vi "ADCP_write_parameter_to_serial_port_emulator_queue.vi"(0 "ADCP In":refnum<class "ADCP.lvclass">, 5 "Parameter Name":string, 7 "Parameter Value":string, 11 "error in (no error)":errorcluster) -> (4 "ADCP out":refnum<class "ADCP.lvclass">, 6 "Queue Out":refnum<queue>, 15 "error out":errorcluster)   [LabVIEW 2017, in "ADCP.lvclass"]
uses:
  ADCP.lvclass
  ADCP.lvclass/ADCP.ctl
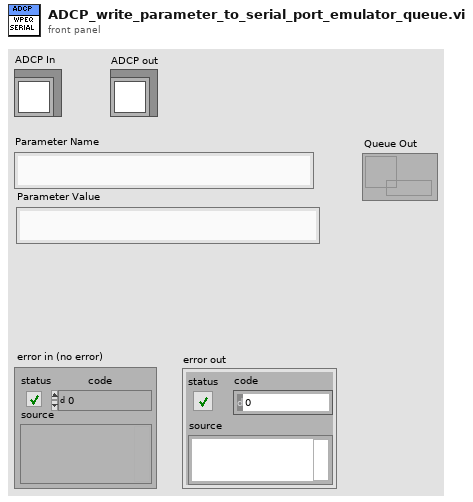
[diagram p1: front panel]
types:
  T1 = typedef "ADCP.lvclass/ADCP_Data_Packet_Transmit_Mode.ctl" = enum16{"Disable", "Single", "Cyclic", "Repeat"}
  T2 = cluster{"Parameters":cluster{"Parameter name":string, "Node name":string, "Node ID":u8, "Frame name":string, "Frame ID":u8, "Start bit":u32, "Bit length":u32, "Factor":dbl, "Offset":dbl, "Minimum":dbl, "Maximum":dbl, "Value":string, "Comments":string, "Data_Type":enum16{"BOOL", "UNSIGNED", "SIGNED", "FLOAT32", "ENUM"}, "Enum List":string[]}[], "Priority":enum16{"LOW", "HIGH"}, "Node name":string, "Node ID":u8, "Frame name":string, "Frame ID":u8, "Data":u32, "Raw bytes":u8[], "Processed bytes":u8[], "Tx count":i32, "Last Tx Time":u32, "Tx interval":u32, "Rx count":i32, "Last Rx Time":u32, "Rx interval":u32, "Tx Enable":bool, "Tx mode":T1, "Repeat/Cyclic Tx interval":u32, "Repeat count":u16}
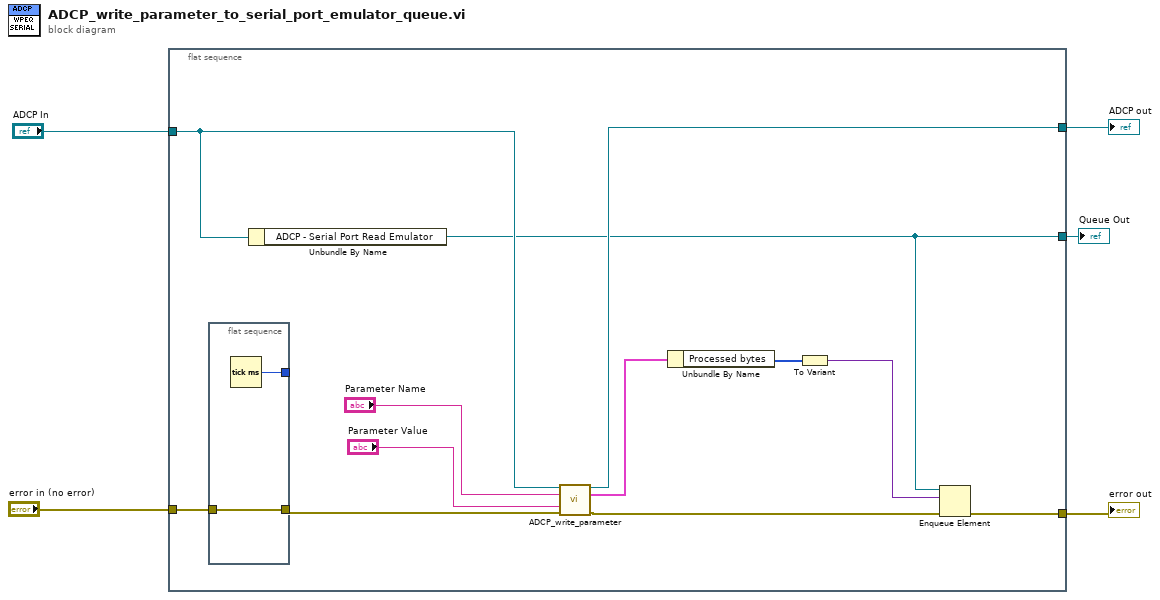
[diagram p0: block diagram]
diagram:
  n1 = flat-sequence {
    tunnel: "ADCP In" -> [w15]
    tunnel: "error in (no error)" -> [w17]
    tunnel: [w8] -> w3
    tunnel: [w7] -> w2
    tunnel: [w6] -> w1
    frame #0 {
      n2 = flat-sequence {
        tunnel: w17 -> [w19]
        tunnel: [w19] -> w16
        tunnel: [w18] -> _
        frame #0 {
          n3 = Tick Count (ms)() -> (millisecond timer value=w18:u32)
        }
      }
      n4 = Unbundle By Name(w15) -> ("ADCP - Serial Port Read Emulator"=w6:refnum<queue>)
      n5 = call "ADCP_write_parameter.vi"("ADCP in"=w15, "Parameter Name"="Parameter Name", "Parameter Value"="Parameter Value", "error in (no error)"=w16) -> ("ADCP out"=w7:refnum<class "ADCP.lvclass">, "Data Packet out"=w12:T2, "error out"=w10:errorcluster)  [unwired: 9 in]
      n6 = Unbundle By Name(w12) -> ("Processed bytes"=w11:u8[])
      n7 = To Variant(anything=w11) -> (Variant=w9:variant)
      n8 = Enqueue Element(queue=w6, element=w9, error in (no error)=w10) -> (error out=w8:errorcluster)  [unwired: 1 in, 2 out]
    }
  }
  "error out" <- w3
  "ADCP out" <- w2
  "Queue Out" <- w1
